vi "Construct Ring Strings Binding.vi"(10 "Ring Refnum":refnum<vi>) -> (0 "error out":errorcluster, 3 "RingStringsBinding":refnum<class "RingStringsBinding.lvclass">)   [LabVIEW 2020, in "MVA Framework.lvlib" / "RingStringsBinding.lvclass"]
doc: "构造下拉列表字符串绑定"
uses:
  RingStringsBinding.lvclass
  RingStringsBinding.lvclass/RingStringsBinding.ctl
  <vilib>/Utility/error.llb/Error Cluster From Error Code.vi
  <vilib>/ErrorRing/Error Ring.xnode
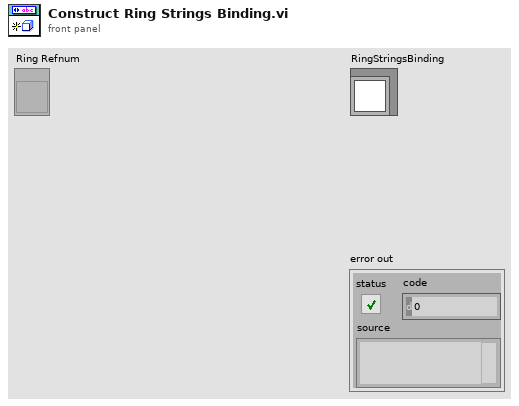
[diagram p1: front panel]
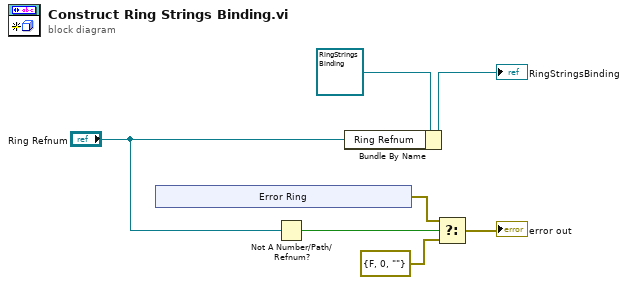
[diagram p0: block diagram]
diagram:
  n1 = xnode "Error Ring"() -> ("error out"=w4:errorcluster)
  n2 = Not A Number/Path/Refnum?(number/path/refnum="Ring Refnum") -> (NaN/Path/Refnum?=w1:bool)
  n3 = Bundle By Name(cluster=refnum<class "RingStringsBinding.lvclass"> refnum ("NamedNumericStringsBinding"), "Ring Refnum"="Ring Refnum") -> (→"RingStringsBinding":refnum<class "RingStringsBinding.lvclass">)
  n4 = Select(t=w4, s=w1, f=errorcluster {"status"=FALSE, "code"=0, "source"=""} ("error constant")) -> (s? t:f=→"error out":errorcluster)
